vi "Copy InstrumentStudio Plug-In Data File.vi"(0 "configuration":T1, 5 "Plugin Library Path":path, 11 "error in":errorcluster) -> (4 "IS Plugin Data File Path":path, 15 "error out":errorcluster)   [LabVIEW 2021, in "InstrumentStudio Plug-In Editor.lvlib"]
uses:
  InstrumentStudio Plug-In Editor.lvlib
  controls/Data Holder.ctl
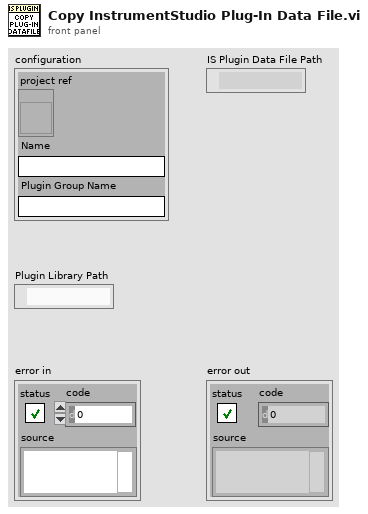
[diagram p1: front panel]
types:
  T1 = typedef "InstrumentStudio Plug-In Editor.lvlib/Data Holder.ctl" = cluster{"project ref":refnum<vi>, "Name":string, "Plugin Group Name":string}
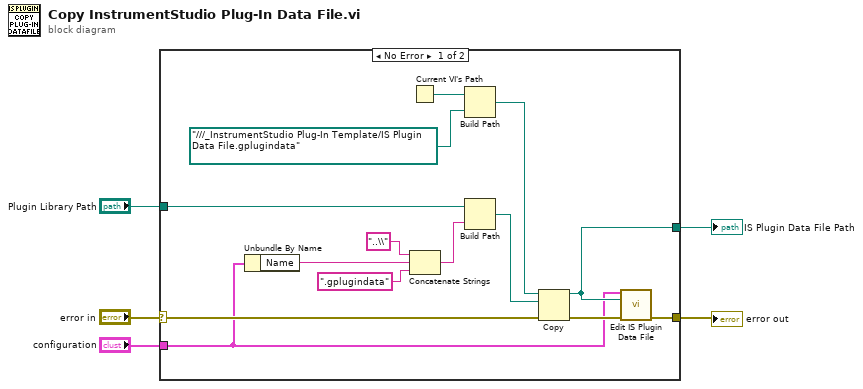
[diagram p0: block diagram]
diagram:
  n1 = case shown="No Error" "error in" {
    selector: "error in" -> [w19 w20]
    tunnel: [w16 w20] -> w5
    tunnel: "Plugin Library Path" -> [w17 _]
    tunnel: "configuration" -> [w8 _]
    tunnel: [w10 _] -> w1
    frame No Error {
      n2 = Unbundle By Name(w8) -> ("Name"=w13:string)
      n3 = Current VI's Path() -> (path=w7:path)
      n4 = Concatenate Strings("..\\" ("string"), w13, ".gplugindata" ("string")) -> (w6:string)
      n5 = Build Path(base path=w7, name or relative path=path "../../../_InstrumentStudio Plug-In Template/IS Plugin Data File.gplugindata") -> (appended path=w14:path)
      n6 = Build Path(base path=w17, name or relative path=w6) -> (appended path=w18:path)
      n7 = Copy(8:w19, 10:w18, 11:w14) -> (0:w15:errorcluster, 3:w10:path)  [unwired: 2 in, 1 out]
      n8 = call "Edit IS Plugin Data File.vi"("configuration"=w8, "Data File Path"=w10, "error in"=w15) -> ("error out"=w16:errorcluster)  [unwired: 12 in]
    }
    frame Error {
    }
  }
  "error out" <- w5
  "IS Plugin Data File Path" <- w1
